vi "Status Byte.vi"(8 "error in (no error)":errorcluster, 11 "VISA resource name":refnum<visa-resource-name>) -> (0 "error out":errorcluster, 1 "Ready":bool, 2 "Enabled":bool, 3 "VISA resource name out":refnum<visa-resource-name>, 4 "TRG Polarity Positive":bool, 5 "Local":bool, 6 "TRG External":bool, 7 "Error number":i8)   [LabVIEW 2020, in "QuPMXdriver.lvlib"]
doc: "Queries the instrument for status byte. Does not generate errors."
uses:
  QuPMXdriver.lvlib
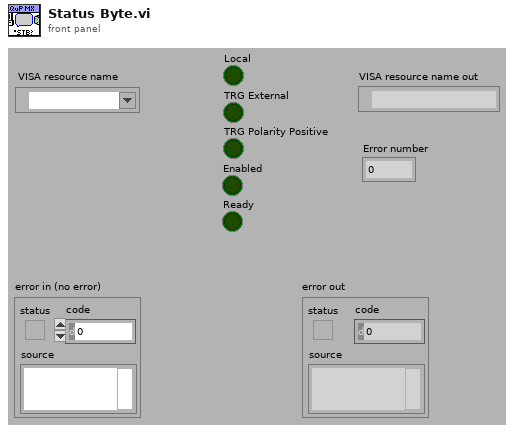
[diagram p1: front panel]
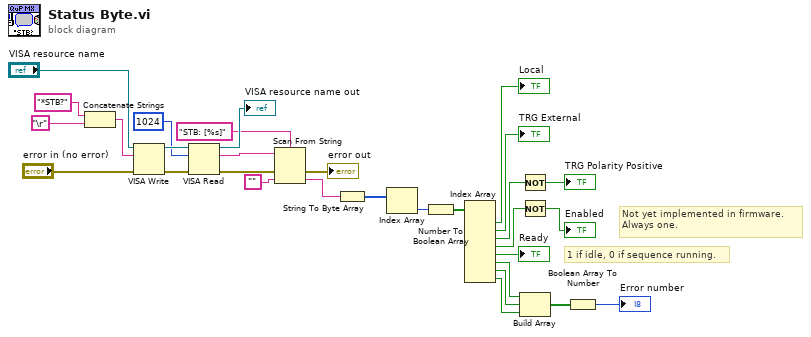
[diagram p0: block diagram]
diagram:
  # "1 if idle, 0 if sequence running."
  # "Not yet implemented in firmware.\nAlways one."
  n1 = Concatenate Strings("*STB?" ("write buffer"), "\r") -> (w12:string)
  n2 = VISA Write(VISA resource name="VISA resource name", write buffer=w12, error in (no error)="error in (no error)") -> (VISA resource name out=w28:refnum<visa-resource-name>, error out=w4:errorcluster)  [unwired: 1 out]
  n3 = VISA Read(VISA resource name=w28, byte count=u32 1024, error in (no error)=w4) -> (VISA resource name out=→"VISA resource name out":refnum<visa-resource-name>, read buffer=w10:string, error out=w3:errorcluster)  [unwired: 1 out]
  n4 = Scan From String(format string="STB: [%s]", input string=w10, error in=w3, default 1="") -> (error out=→"error out":errorcluster, output 1=w9:string)  [unwired: 1 in, 2 out]
  n5 = String To Byte Array(string=w9) -> (unsigned byte array=w23:u8[])
  n6 = Index Array(array=w23) -> (element=w22:u8)  [unwired: 1 in]
  n7 = Number To Boolean Array(number=w22) -> (Boolean array=w25:bool[])
  n8 = Index Array(array=w25) -> (element #1=→"Local":bool, element #2=→"TRG External":bool, element #3=w8:bool, element #4=w5:bool, element #5=→"Ready":bool, element #6=w19:bool, element #7=w18:bool, element #8=w17:bool)  [unwired: 8 in]
  n9 = Not(x=w8) -> (.not. x?=→"TRG Polarity Positive":bool)
  n10 = Not(x=w5) -> (.not. x?=→"Enabled":bool)
  n11 = Build Array(w19, w18, w17) -> (w16:bool[])
  n12 = Boolean Array To Number(Boolean array=w16) -> (number=→"Error number":u32)
